vi "Handle Error.vi"(8 "error in (no error)":errorcluster, 11 "Primitive in":refnum<class "Primitive.lvclass">) -> (0 "error out":errorcluster, 2 "stop actor?":bool=TRUE, 3 "Primitive out":refnum<class "Primitive.lvclass">)   [LabVIEW 2025, in "Primitive.lvlib" / "Primitive.lvclass"]
doc: "<p>(<strong>Filename</strong>: <span class=\"dnl\">Actor Framework.lvlib:Actor.lvclass:Handle Error.vi</span>)</p>\n<p>Defines how the actor handles an error that occurred while processing a message. By default, this method does nothing except stop the actor.</p>"
uses:
  Primitive.lvclass
  Primitive.lvclass/Primitive.ctl
  <vilib>/MGI/Monitored Actor/Monitored Actor/Monitored Actor/Monitored Actor.lvclass
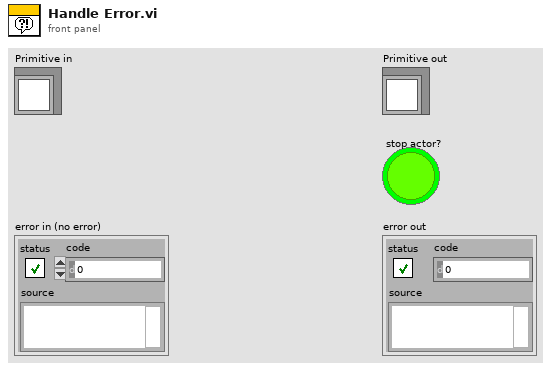
[diagram p1: front panel]
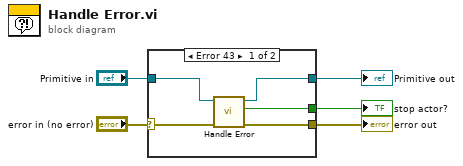
[diagram p0: block diagram]
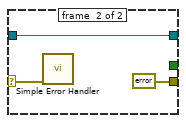
[diagram p2: hidden frame]
diagram:
  n1 = case shown="Error 43" "error in (no error)" {
    selector: "error in (no error)" -> [w7 w11]
    tunnel: [w10 errorcluster {"status"=FALSE, "code"=0, "source"=""} ("error out")] -> w4
    tunnel: [w9 _] -> w5
    tunnel: [w8 w13] -> w1
    tunnel: "Primitive in" -> [w6 w13]
    frame #0 {
      n2 = call-parent "Handle Error.vi"("error in (no error)"=w7, "Actor in"=w6) -> ("error out"=w10:errorcluster, "stop actor?"=w9:bool, "Actor out"=w8:refnum<class "Primitive.lvclass">)  [unwired: 7 in]
    }
    frame #1 {
      n3 = call <vilib>:"Simple Error Handler.vi"("error in (no error)"=w11) -> ()  [unwired: 4 in, 5 out]
    }
  }
  "Primitive out" <- w1
  "error out" <- w4
  "stop actor?" <- w5
